vi "五参数标样核查.vi"(11 "启动参数":T1={"测量模式"=enum."水样测试", "数据标记表"="N", "输出参数"={"水温"=FALSE, "pH"=FALSE, "DO"=FALSE, "浊度"=FALSE, "电导率"=FALSE, "保存组数"=0.0}}) -> ()   [LabVIEW 2016, in "斯坦道仪器.lvlib"]
uses:
  PLC/PLC.lvlib
panel:
  out "枚举":T2(ring)
  out "状态":string
  out "数值":i32
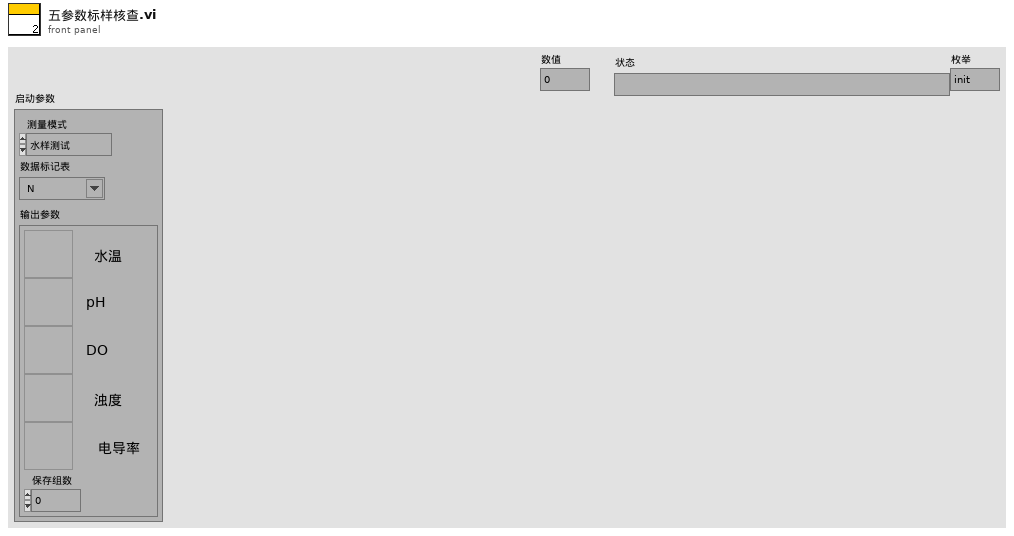
[diagram p1: front panel]
types:
  T1 = cluster{"测量模式":enum16{"待机", "水样测试", "标样核查", "零点核查", "跨度核查", "空白测试", "平行样测试", "加标回收", "空白校准", "标样校准", "初始化（清洗）"}, "数据标记表":string, "输出参数":cluster{"水温":bool, "pH":bool, "DO":bool, "浊度":bool, "电导率":bool, "保存组数":dbl}}
  T2 = enum16{"init", "开机", "启动测量", "读取测量值", "存储数据", "关闭测量", "关机", "结束"}
  T3 = cluster{"时间标识":timestamp, "设备":string, "日志信息":string, "流程参数":string}
  T4 = cluster{"starting address":u16, "holding register value":u16}
  T5 = enum16{"idle", "init", "读状态", "读参数", "多个写入", "单个写入", "线圈写入"}
  T6 = enum16{"待机", "水样测试", "标样核查", "零点核查", "跨度核查", "空白测试", "平行样测试", "加标回收", "空白校准", "标样校准", "初始化（清洗）"}
  T7 = cluster{"数据标记表":string, "测量模式":enum16{"待机", "水样测试", "标样核查", "零点核查", "跨度核查", "空白测试", "平行样测试", "加标回收", "空白校准", "标样校准", "初始化（清洗）"}, "database":string}
  T8 = cluster{"因子编码":string, "单位":string, "标样参考值":sgl, "水样数据时间":timestamp, "水样实测值":sgl, "水样数据标识":string, "K":sgl, "B":sgl, "T":sgl, "H":sgl, "水深":sgl}
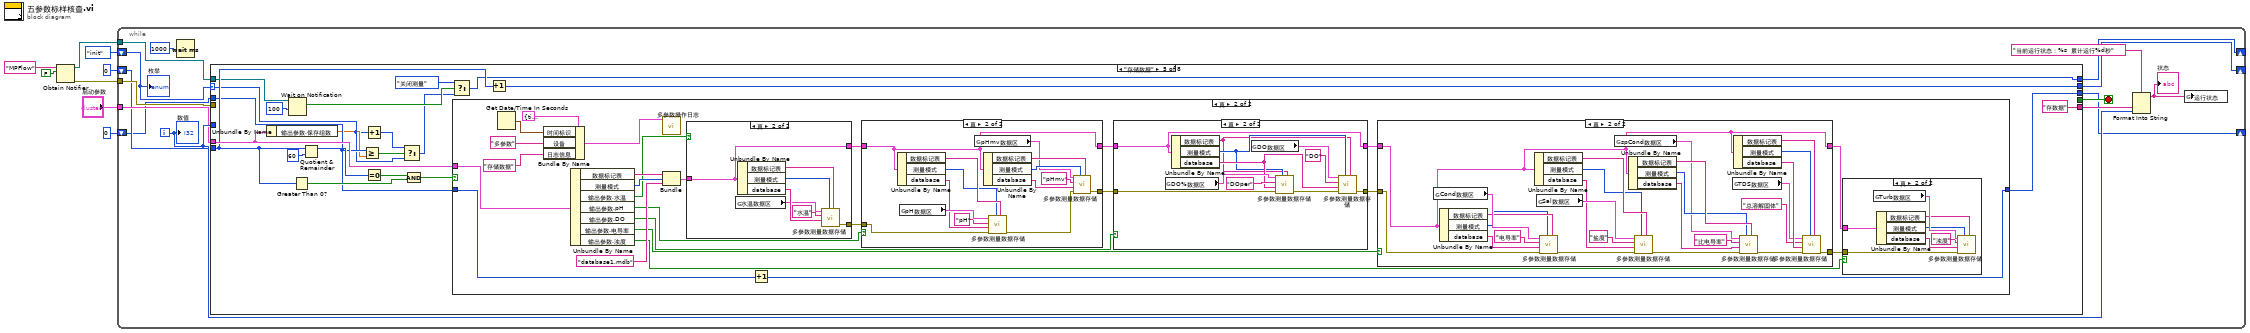
[diagram p0: block diagram]
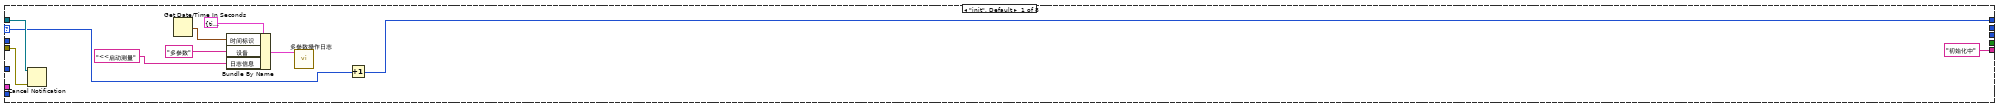
[diagram p2: hidden frame]
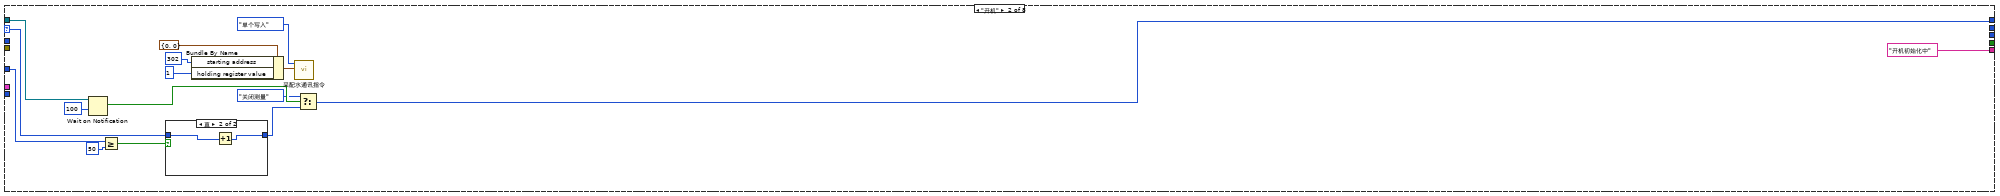
[diagram p3: hidden frame]
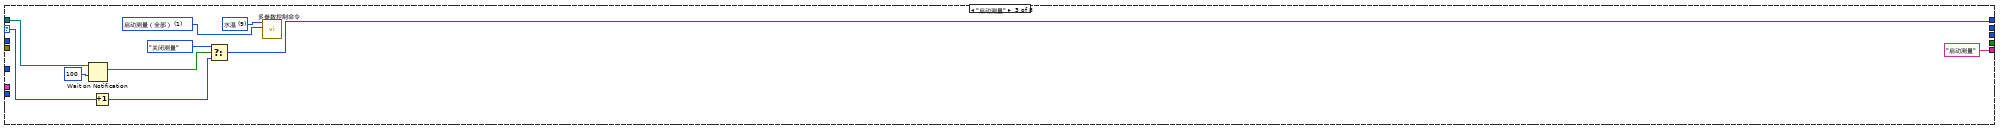
[diagram p5: hidden frame]
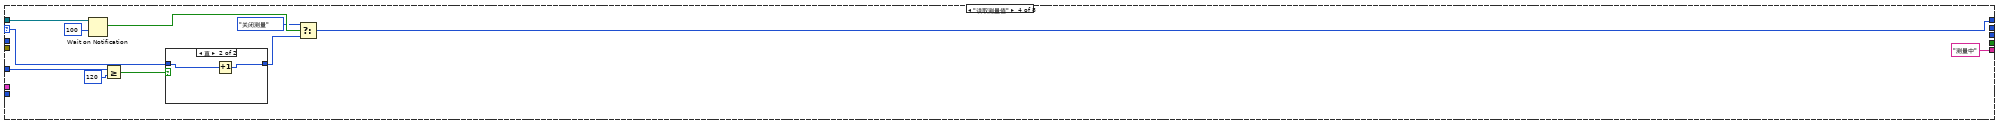
[diagram p6: hidden frame]
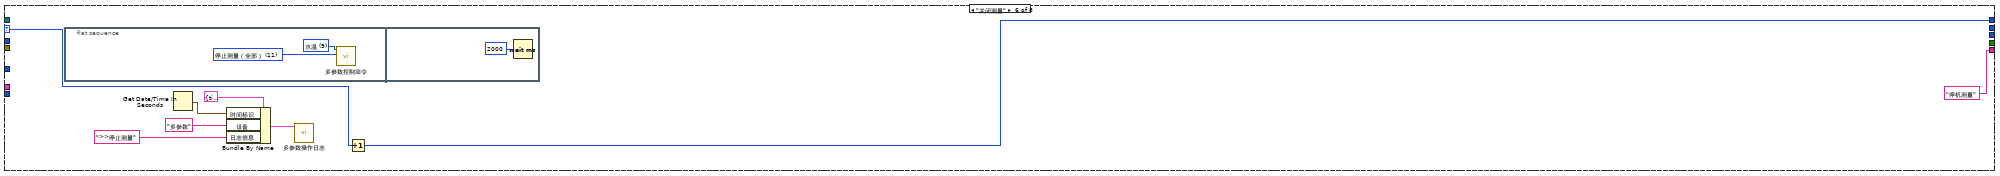
[diagram p14: hidden frame]
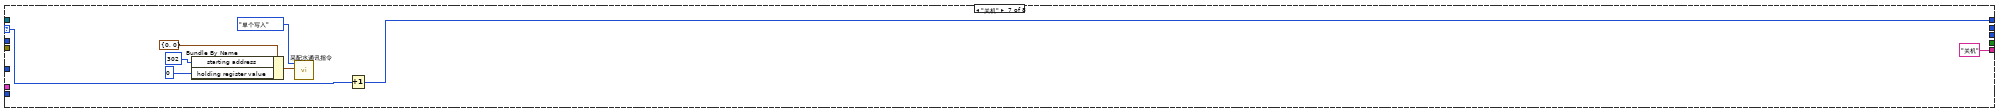
[diagram p15: hidden frame]
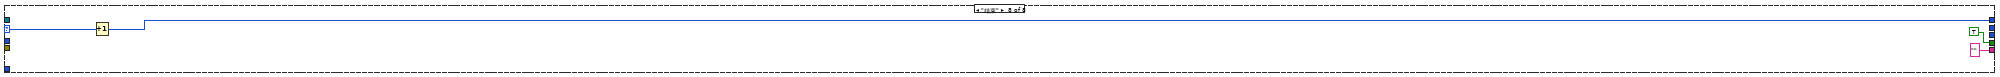
[diagram p16: hidden frame]
diagram:
  n1 = Obtain Notifier(name (unnamed)="MPFlow" ("名称（未命名）"), notification data type=FALSE) -> (notifier out=w5:refnum<notifier>, error out=w4:errorcluster)  [unwired: 2 in, 1 out]
  n2 = while {
    shift-right: [w19] -> _
    shift-left: T2."init" ("枚举") -> [w23]
    tunnel: w5 -> [w21]
    tunnel: w4 -> [w20]
    tunnel: "启动参数" -> [w13]
    shift-right: [w11] -> _
    shift-left: u32 0 ("等待时间（毫秒）") -> [w12]
    shift-right: [w9] -> _
    shift-left: u32 0 ("等待时间（毫秒）") -> [w10]
    i -> [w15]
    stop <- w22 stop-if-true
    n3 = Wait (ms)(milliseconds to wait=u32 1000 ("等待时间（毫秒）")) -> ()  [unwired: 1 out]
    n4 = case shown="\"存储数据\"" w23 {
      selector: w23 -> [w31 w44 w62 w73 w77 w200 w206 w214]
      tunnel: [_ _ _ _ _ _ _ TRUE] -> w22
      tunnel: w21 -> [w33 w39 w61 w70 w87 _ _ _]
      tunnel: w20 -> [w32 _ _ _ _ _ _ _]
      tunnel: [w30 w37 w58 w68 w83 w199 w205 w213] -> w19
      tunnel: w15 -> [_ w43 _ w63 _ _ _ _]
      tunnel: ["初始化中" ("状态") "开机初始化中" ("状态") "启动测量" ("状态") "测量中" ("状态") "存数据" ("状态") "停机测量" ("状态") "关机" ("状态") "" ("状态")] -> w16
      tunnel: w13 -> [_ _ _ _ w96 _ _ _]
      tunnel: w12 -> [_ _ _ _ w90 _ _ _]
      tunnel: [_ _ _ _ w91 _ _ _] -> w11
      tunnel: w10 -> [_ _ _ _ w80 _ _ _]
      tunnel: [_ _ _ _ w82 _ _ _] -> w9
      frame "init", Default {
        n5 = Cancel Notification(0:w33, 3:w32) -> ()  [unwired: 3 out]
        n6 = Get Date/Time In Seconds() -> (seconds since 1Jan1904=w27:timestamp)
        n7 = Bundle By Name(cluster=T3 {"时间标识"=timestamp(0 s since 1904-01-01), "设备"="", "日志信息"="", "流程参数"=""} ("data in"), "时间标识"=w27, "设备"="多参数", "日志信息"="<<启动测量") -> (w26:T3)
        n8 = call "多参数操作日志.vi"("data in"=w26) -> ()  [unwired: 10 in, 1 out]
        n9 = Increment(x=w31) -> (x+1=w30:T2)
      }
      frame "开机" {
        n10 = Wait on Notification(notifier=w39, timeout in ms (-1)=100 ("超时毫秒(-1)")) -> (notification=w40:bool)  [unwired: 2 in, 3 out]
        n11 = Greater Or Equal?(x=w43, y=50) -> (x >= y?=w41:bool)
        n12 = case shown="真" w41 {
          tunnel: w44 -> [w50 w52]
          tunnel: [w50 w51] -> w38
          frame False {
          }
          frame True {
            n13 = Increment(x=w52) -> (x+1=w51:T2)
          }
        }
        n14 = Bundle By Name(cluster=T4 {"starting address"=0, "holding register value"=0}, "starting address"=u16 302, "holding register value"=u16 1) -> (w47:T4)
        n15 = call "采配水通讯指令.vi"("数据"=w47, "命令"=T5."单个写入") -> ()  [unwired: 10 in]
        n16 = Select(t=T2."关闭测量" ("枚举"), s=w40, f=w38) -> (s? t:f=w37:T2)
      }
      frame "启动测量" {
        w53 = u16 1 items=["启动测量（全部）"=1, "初始化（清洗）"=10, "停止测量（全部）"=11, "校时"=13, "启动测量（单个传感器）"=19, "停止测量（单个传感器）"=20] ("控制命令")
        w54 = u16 9 items=["氨氮"=3, "水温"=9, "pH值"=10, "溶解氧"=11, "电导率"=12, "浊度"=13, "叶绿素a"=14, "藻密度"=15, "蓝绿藻"=16, "氧化还原电位"=17, "溶解氧%"=18, "盐度"=19] ("站号")
        n17 = Wait on Notification(notifier=w61, timeout in ms (-1)=100 ("超时毫秒(-1)")) -> (notification=w60:bool)  [unwired: 2 in, 3 out]
        n18 = Increment(x=w62) -> (x+1=w59:T2)
        n19 = Select(t=T2."关闭测量" ("枚举"), s=w60, f=w59) -> (s? t:f=w58:T2)
        n20 = call "多参数控制命令.vi"("控制命令"=w53, "站号"=w54) -> ()  [unwired: 9 in, 1 out]
      }
      frame "读取测量值" {
        n21 = Wait on Notification(notifier=w70, timeout in ms (-1)=100 ("超时毫秒(-1)")) -> (notification=w71:bool)  [unwired: 2 in, 3 out]
        n22 = Greater Or Equal?(x=w63, y=120) -> (x >= y?=w72:bool)
        n23 = case shown="真" w72 {
          tunnel: w73 -> [w74 w76]
          tunnel: [w74 w75] -> w69
          frame False {
          }
          frame True {
            n24 = Increment(x=w76) -> (x+1=w75:T2)
          }
        }
        n25 = Select(t=T2."关闭测量" ("枚举"), s=w71, f=w69) -> (s? t:f=w68:T2)
      }
      frame "存储数据" {
        n26 = Unbundle By Name(w96) -> ("输出参数.保存组数"=w79:dbl)
        n27 = Wait on Notification(notifier=w87, timeout in ms (-1)=100 ("超时毫秒(-1)")) -> (notification=w86:bool)  [unwired: 2 in, 3 out]
        n28 = Greater Than 0?(x=w90) -> (x > 0?=w89:bool)
        n29 = Quotient & Remainder(x=w90, y=u32 60) -> (x-y*floor(x/y)=w94:u32)  [unwired: 1 out]
        n30 = Greater Or Equal?(x=w80, y=w79) -> (x >= y?=w81:bool)
        n31 = Increment(x=w77) -> (x+1=w78:T2)
        n32 = Equal To 0?(x=w94) -> (x = 0?=w93:bool)
        n33 = Select(t=w78, s=w81, f=w77) -> (s? t:f=w85:T2)
        n34 = Compound Arithmetic op=AND ("复合运算")(w93, w89) -> (w92:bool)
        n35 = Select(t=T2."关闭测量", s=w86, f=w85) -> (s? t:f=w83:T2)
        n36 = case shown="真" w92 {
          tunnel: w96 -> [_ w123]
          tunnel: w80 -> [w98 w100]
          tunnel: [w98 w99] -> w82
          frame False {
          }
          frame True {
            n37 = Get Date/Time In Seconds() -> (seconds since 1Jan1904=w109:timestamp)
            n38 = Bundle By Name(cluster=T3 {"时间标识"=timestamp(0 s since 1904-01-01), "设备"="", "日志信息"="", "流程参数"=""} ("data in"), "时间标识"=w109, "设备"="多参数", "日志信息"="存储数据") -> (w108:T3)
            n39 = Unbundle By Name(w123) -> ("数据标记表"=w117:string, "测量模式"=w116:T6, "输出参数.水温"=w105:bool, "输出参数.pH"=w104:bool, "输出参数.DO"=w103:bool, "输出参数.电导率"=w102:bool, "输出参数.浊度"=w101:bool)
            n40 = call "多参数操作日志.vi"("data in"=w108) -> ()  [unwired: 10 in, 1 out]
            n41 = Bundle("数据标记表"=w117, "测量模式"=w116, "database"="database1.mdb") -> (w115:T7)  [unwired: 1 in]
            n42 = case shown="真" w105 {
              tunnel: [_ w191] -> w122
              tunnel: w115 -> [w185 w190]
              tunnel: [w185 w190] -> w114
              frame False {
              }
              frame True {
                n43 = global read "多参数全局变量.vi" "水温数据区"() -> (w186:T8)
                n44 = Unbundle By Name(w190) -> ("数据标记表"=w189:string, "测量模式"=w188:T6, "database"=w187:string)
                n45 = call "多参数测量数据存储.vi"("数据标记表"=w189, "测量模式"=w188, "database"=w187, "table输入"="水温", "data in"=w186) -> ("error out"=w191:errorcluster)  [unwired: 6 in]
              }
            }
            n46 = Increment(x=w100) -> (x+1=w99:u32)
            n47 = case shown="真" w104 {
              tunnel: w122 -> [_ w184]
              tunnel: [_ w173] -> w121
              tunnel: w114 -> [w170 w178]
              tunnel: [w170 w178] -> w112
              frame False {
              }
              frame True {
                n48 = Unbundle By Name(w178) -> ("数据标记表"=w181:string, "测量模式"=w180:T6, "database"=w179:string)
                n49 = global read "多参数全局变量.vi" "pH数据区"() -> (w183:T8)
                n50 = global read "多参数全局变量.vi" "pHmv数据区"() -> (w172:T8)
                n51 = Unbundle By Name(w178) -> ("数据标记表"=w177:string, "测量模式"=w176:T6, "database"=w175:string)
                n52 = call "多参数测量数据存储.vi"("数据标记表"=w181, "测量模式"=w180, "error in (no error)"=w184, "database"=w179, "table输入"="pH", "data in"=w183) -> ("error out"=w174:errorcluster)  [unwired: 5 in]
                n53 = call "多参数测量数据存储.vi"("数据标记表"=w177, "测量模式"=w176, "error in (no error)"=w174, "database"=w175, "table输入"="pHmv", "data in"=w172) -> ("error out"=w173:errorcluster)  [unwired: 5 in]
              }
            }
            n54 = case shown="真" w103 {
              tunnel: w121 -> [_ w169]
              tunnel: [_ w165] -> w120
              tunnel: [w158 w162] -> w113
              tunnel: w112 -> [w158 w162]
              frame False {
              }
              frame True {
                n55 = global read "多参数全局变量.vi" "DO%数据区"() -> (w164:T8)
                n56 = Unbundle By Name(w162) -> ("数据标记表"=w159:string, "测量模式"=w160:T6, "database"=w161:string)
                n57 = global read "多参数全局变量.vi" "DO数据区"() -> (w166:T8)
                n58 = call "多参数测量数据存储.vi"("数据标记表"=w159, "测量模式"=w160, "error in (no error)"=w169, "database"=w161, "table输入"="DOper", "data in"=w164) -> ("error out"=w168:errorcluster)  [unwired: 5 in]
                n59 = call "多参数测量数据存储.vi"("数据标记表"=w159, "测量模式"=w160, "error in (no error)"=w168, "database"=w161, "table输入"="DO", "data in"=w166) -> ("error out"=w165:errorcluster)  [unwired: 5 in]
              }
            }
            n60 = case shown="真" w102 {
              tunnel: w120 -> [_ w155]
              tunnel: [_ w136] -> w119
              tunnel: w113 -> [w131 w145]
              tunnel: [w131 w145] -> w111
              frame False {
              }
              frame True {
                n61 = global read "多参数全局变量.vi" "Cond数据区"() -> (w157:T8)
                n62 = Unbundle By Name(w145) -> ("数据标记表"=w150:string, "测量模式"=w149:T6, "database"=w151:string)
                n63 = Unbundle By Name(w145) -> ("数据标记表"=w148:string, "测量模式"=w147:T6, "database"=w146:string)
                n64 = global read "多参数全局变量.vi" "Sal数据区"() -> (w153:T8)
                n65 = call "多参数测量数据存储.vi"("数据标记表"=w150, "测量模式"=w149, "error in (no error)"=w155, "database"=w151, "table输入"="电导率", "data in"=w157) -> ("error out"=w154:errorcluster)  [unwired: 5 in]
                n66 = global read "多参数全局变量.vi" "spCond数据区"() -> (w135:T8)
                n67 = Unbundle By Name(w145) -> ("数据标记表"=w144:string, "测量模式"=w143:T6, "database"=w142:string)
                n68 = call "多参数测量数据存储.vi"("数据标记表"=w148, "测量模式"=w147, "error in (no error)"=w154, "database"=w146, "table输入"="盐度", "data in"=w153) -> ("error out"=w141:errorcluster)  [unwired: 5 in]
                n69 = global read "多参数全局变量.vi" "TDS数据区"() -> (w134:T8)
                n70 = Unbundle By Name(w145) -> ("数据标记表"=w137:string, "测量模式"=w138:T6, "database"=w139:string)
                n71 = call "多参数测量数据存储.vi"("数据标记表"=w144, "测量模式"=w143, "error in (no error)"=w141, "database"=w142, "table输入"="比电导率", "data in"=w135) -> ("error out"=w140:errorcluster)  [unwired: 5 in]
                n72 = call "多参数测量数据存储.vi"("数据标记表"=w137, "测量模式"=w138, "error in (no error)"=w140, "database"=w139, "table输入"="总溶解固体", "data in"=w134) -> ("error out"=w136:errorcluster)  [unwired: 5 in]
              }
            }
            n73 = case shown="真" w101 {
              tunnel: w119 -> [_ w130]
              tunnel: w111 -> [_ w127]
              frame False {
              }
              frame True {
                n74 = global read "多参数全局变量.vi" "Turb数据区"() -> (w129:T8)
                n75 = Unbundle By Name(w127) -> ("数据标记表"=w124:string, "测量模式"=w125:T6, "database"=w126:string)
                n76 = call "多参数测量数据存储.vi"("数据标记表"=w124, "测量模式"=w125, "error in (no error)"=w130, "database"=w126, "table输入"="浊度", "data in"=w129) -> ()  [unwired: 5 in, 1 out]
              }
            }
          }
        }
        n77 = Increment(x=w90) -> (x+1=w91:u32)
      }
      frame "关闭测量" {
        n78 = flat-sequence {
          frame #0 {
            w201 = u16 11 items=["启动测量（全部）"=1, "初始化（清洗）"=10, "停止测量（全部）"=11, "校时"=13, "启动测量（单个传感器）"=19, "停止测量（单个传感器）"=20] ("控制命令")
            w202 = u16 9 items=["氨氮"=3, "水温"=9, "pH值"=10, "溶解氧"=11, "电导率"=12, "浊度"=13, "叶绿素a"=14, "藻密度"=15, "蓝绿藻"=16, "氧化还原电位"=17, "溶解氧%"=18, "盐度"=19] ("站号")
            n79 = call "多参数控制命令.vi"("控制命令"=w201, "站号"=w202) -> ()  [unwired: 9 in, 1 out]
          }
          frame #1 {
            n80 = Wait (ms)(milliseconds to wait=u32 2000 ("等待时间（毫秒）")) -> ()  [unwired: 1 out]
          }
        }
        n81 = Get Date/Time In Seconds() -> (seconds since 1Jan1904=w196:timestamp)
        n82 = Bundle By Name(cluster=T3 {"时间标识"=timestamp(0 s since 1904-01-01), "设备"="", "日志信息"="", "流程参数"=""} ("data in"), "时间标识"=w196, "设备"="多参数", "日志信息"=">>停止测量") -> (w195:T3)
        n83 = call "多参数操作日志.vi"("data in"=w195) -> ()  [unwired: 10 in, 1 out]
        n84 = Increment(x=w200) -> (x+1=w199:T2)
      }
      frame "关机" {
        n85 = Bundle By Name(cluster=T4 {"starting address"=0, "holding register value"=0}, "starting address"=u16 302, "holding register value"=u16 0) -> (w209:T4)
        n86 = call "采配水通讯指令.vi"("数据"=w209, "命令"=T5."单个写入") -> ()  [unwired: 10 in]
        n87 = Increment(x=w206) -> (x+1=w205:T2)
      }
      frame "结束" {
        n88 = Increment(x=w214) -> (x+1=w213:T2)
      }
    }
    n89 = Format Into String(format string="当前运行状态：%s  累计运行%d秒" ("格式字符串"), w16, w15) -> (resulting string=w14:string)  [unwired: 2 in, 1 out]
    "状态" <- w14
    n90 = global write "多参数全局变量.vi" "运行状态"(w14) -> ()
    "数值" <- w15
    "枚举" <- w23
  }
